vi "MultipleUserEvent.vi"() -> ()   [LabVIEW 2011]
uses:
  <vilib>/Platform/TimedLoop/XDataNode/timing_clust.ctl
  <vilib>/Platform/TimedLoop/XDataNode/nitl_modes.ctl
  <vilib>/Platform/TimedLoop/XDataNode/wakeup.ctl
  <vilib>/Platform/TimedLoop/XDataNode/XDataNode.xnode
  <vilib>/Platform/TimedLoop/XDataNode/XDNodeRunTimeDep.lvlib
panel:
  out "Time Stamp":timestamp
  out "采样次数":string
  out "Waveform Chart":dbl(graph)
  in  "stop":bool
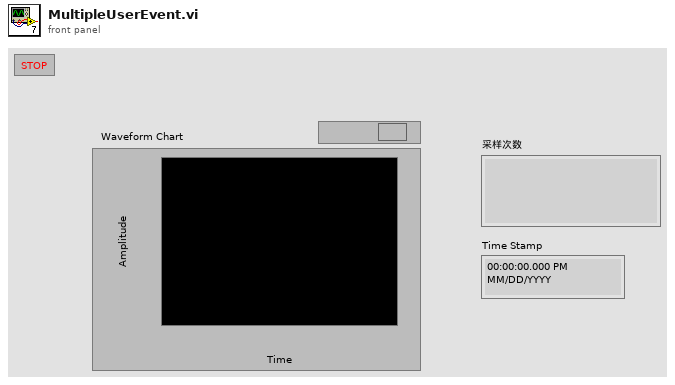
[diagram p1: front panel]
types:
  T1 = typedef "XDNodeRunTimeDep.lvlib/timing_clust.ctl" = cluster{"Expected End [f-1]":u64, "Actual End [f-1]":u64, "Finished Late? [f-1]":bool, "Expected End [i-1]":u64, "Actual End [i-1]":u64, "Finished Late? [i-1]":bool, "Expected Start [i]":u64, "Actual Start [i]":u64, "Expected Start [f]":u64, "Actual Start [f]":u64, "Source Name":string, "Structure Name":string, "Period":i64, "Deadline":i64, "Offset":i64, "Start":i64, "Priority":i32, "Timeout":i32, "Mode":T2, "Wakeup Reason":T3, "Error":errorcluster, "Source Type":string, "Secondary Source Type":string, "Global End Time":u64, "Global Start Time":u64, "Frame Duration":u64, "Iteration Duration":u64, "Assigned CPU":i32, "I/O Scan Engine Mode":u32}
  T2 = typedef "XDNodeRunTimeDep.lvlib/nitl_modes.ctl" = enum32{"No Change", "Process missed periods, maintain original phase", "Discard missed periods, maintain original phase", "Process missed periods, ignore original phase", "Discard missed periods, ignore original phase"}
  T3 = typedef "XDNodeRunTimeDep.lvlib/wakeup.ctl" = enum32{"Normal", "Aborted", "Asynchronous wakeup", "Timing source error", "Timed loop error", "Timeout"}
  T4 = cluster{"data":refnum<user-event>, "count":refnum<user-event>}
  T5 = cluster{"seconds since 1Jan1904":timestamp, "number: 0 to 1":dbl}
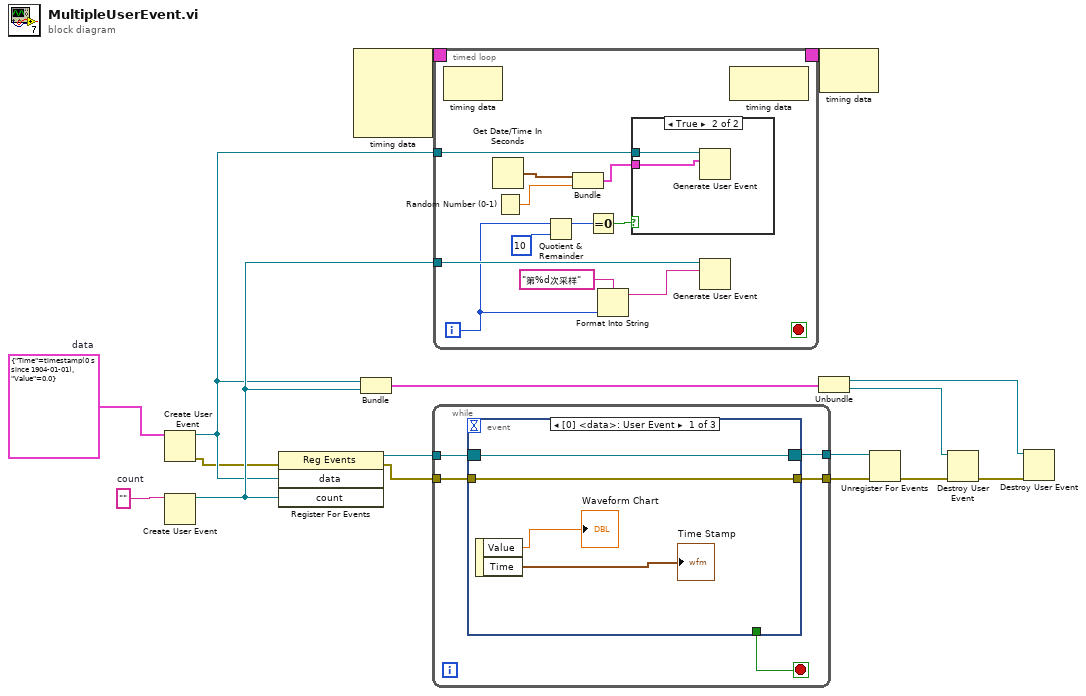
[diagram p0: block diagram]
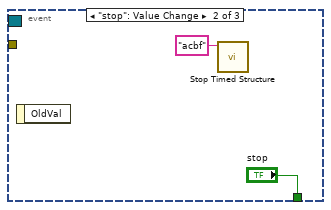
[diagram p3: hidden frame]
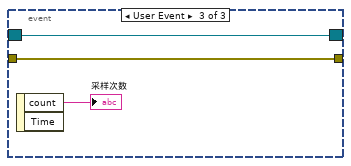
[diagram p4: hidden frame]
diagram:
  w12 = ""  # count
  w14 = cluster{"Time":timestamp, "Value":dbl} {"Time"=timestamp(0 s since 1904-01-01), "Value"=0.0}  # data
  n1 = Create User Event(user event datatype=w14) -> (user event=w5:refnum<user-event>, error out=w1:errorcluster)  [unwired: 1 in]
  n2 = Create User Event(user event datatype=w12) -> (user event=w6:refnum<user-event>)  [unwired: 1 in, 1 out]
  n3 = register-events(error in=w1, w5, w6) -> (reference out=w13:refnum<event-registration>, error out=w11:errorcluster)  [unwired: 1 in]
  n4 = node-c288() -> (w16:T1)  [unwired: 4 in]
  n5 = Bundle("data"=w5, "count"=w6) -> (w4:T4)  [unwired: 1 in]
  n6 = while {
    tunnel: w13 -> [w21]
    tunnel: w11 -> [w20]
    tunnel: [w19] -> w10
    tunnel: [w18] -> w9
    stop <- w17 stop-if-true
    n7 = event shown="[0] <data>: User Event" {
      selector: w21 -> [w25 _ w29]
      dyn-events: [w25 _ w29] -> w19
      timeout: _ -> [_ _ _]
      tunnel: [w24 _ w28] -> w18
      tunnel: w20 -> [w24 _ w28]
      tunnel: [_ "stop" _] -> w17
      event User Event {
        n8 = event-data() -> ("Value"=→"Waveform Chart":dbl, "Time"=→"Time Stamp":timestamp)  [unwired: 1 in]
      }
      event "stop": Value Change {
        n9 = event-data() -> ()  [unwired: 1 in, 1 out]
        n10 = call <vilib>:"Stop Timed Structure.vi"("name"="acbf") -> ()  [unwired: 10 in, 1 out]
      }
      event User Event {
        n11 = event-data() -> ("count"=→"采样次数":string)  [unwired: 1 in, 1 out]
      }
    }
  }
  n12 = timed-loop {
    timing: w16 -> [_]
    timing-out: [_] -> w15
    tunnel: w5 -> [w31]
    tunnel: w6 -> [w41]
    i -> [w37]
    stop <- _ stop-if-true
    n13 = node-c288() -> ()  [unwired: 1 in, 1 out]
    n14 = Get Date/Time In Seconds() -> (seconds since 1Jan1904=w34:timestamp)
    n15 = Random Number (0-1)() -> (number: 0 to 1=w33:dbl)
    n16 = Quotient & Remainder(x=w37, y=10) -> (x-y*floor(x/y)=w35:i32)  [unwired: 1 out]
    n17 = Bundle("seconds since 1Jan1904"=w34, "number: 0 to 1"=w33) -> (w32:T5)  [unwired: 1 in]
    n18 = Equal To 0?(x=w35) -> (x = 0?=w36:bool)
    n19 = Format Into String(format string="第%d次采样", w37) -> (resulting string=w39:string)  [unwired: 2 in, 1 out]
    n20 = case shown="True" w36 {
      tunnel: w32 -> [_ w42]
      tunnel: w31 -> [_ w43]
      frame False {
      }
      frame True {
        n21 = Generate User Event(user event=w43, event data cluster=w42) -> ()  [unwired: 1 in, 2 out]
      }
    }
    n22 = Generate User Event(user event=w41, event data cluster=w39) -> ()  [unwired: 1 in, 2 out]
    n23 = node-c288() -> ()  [unwired: 1 in, 1 out]
  }
  n24 = Unbundle(w4) -> ("data"=w2:refnum<user-event>, "count"=w3:refnum<user-event>)
  n25 = node-c288(w15) -> ()  [unwired: 1 out]
  n26 = Unregister For Events(event registration refnum=w10, error in=w9) -> (error out=w8:errorcluster)
  n27 = Destroy User Event(user event=w3, error in=w8) -> (error out=w7:errorcluster)
  n28 = Destroy User Event(user event=w2, error in=w7) -> ()  [unwired: 1 out]
